vi "WaitForMoveComplete.vi"(6 "timeout (5000 ms)":i32=5000, 8 "error in (no error)":errorcluster, 11 "XYStage":refnum<class "XYStage.lvclass">) -> (0 "error out":errorcluster, 2 "move complete":bool, 3 "XYStage out":refnum<class "XYStage.lvclass">)   [LabVIEW 2013, in "XYStage.lvclass"]
doc: "---------------------------------------------------------------\nJKI State Machine Objects™\nhttp://jki.net/state-machine-objects/\nCopyright (C) 2005-2015, JKI <info@jki.net>\nALL RIGHTS RESERVEDJKI State Machine Objects (SMO) 1.0.0.4\nJKI - JKI\nCopyright (c) 2015, JKI"
uses:
  XYStage.lvclass
  <vilib>/JKI/JKI SMO/SMO/SMO.lvclass
  <vilib>/JKI/JKI SMO/SMO/Typedefs/SMOState --Enum.ctl
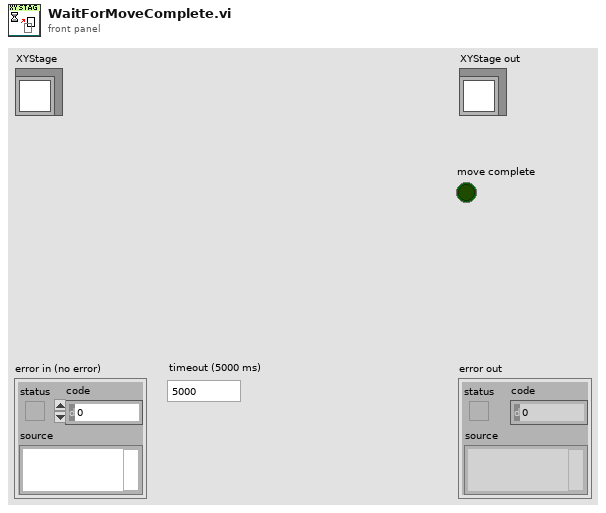
[diagram p1: front panel]
types:
  T1 = typedef "SMO.lvclass/Protected Events.ctl" = cluster{"StopProcesses":refnum<user-event>, "AbortProcesses":refnum<user-event>, "Config Changed":refnum<user-event>}
  T2 = typedef "SMO.lvclass/Public Events.ctl" = cluster{"Error":refnum<user-event>, "State":refnum<user-event>}
  T3 = typedef "XYStage.lvclass/PublicEvents--Cluster.ctl" = cluster{"MoveComplete":refnum<user-event>, "NewPosition":refnum<user-event>, "UpdatedNamedPosition":refnum<user-event>, "MoveStarted":refnum<user-event>}
  T4 = typedef "SMO.lvclass/SMOState --Enum.ctl" = enum16{"unknown", "Created", "Started", "Stopped"}
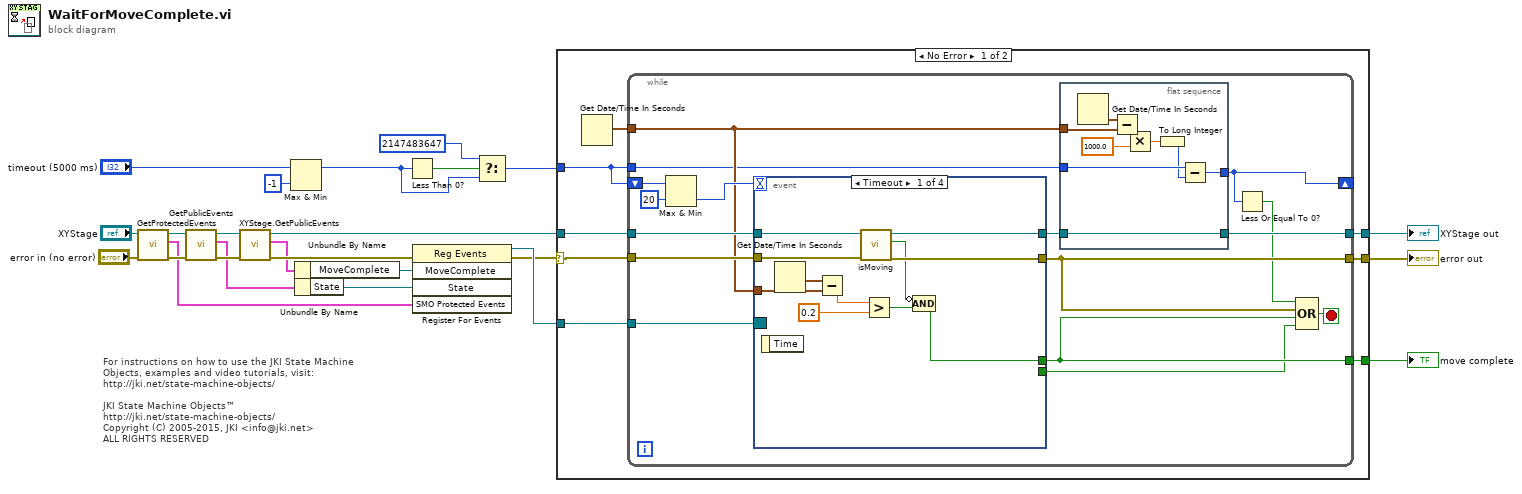
[diagram p0: block diagram]
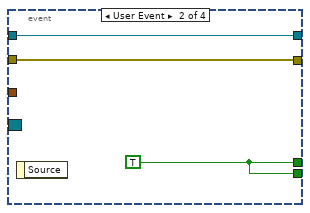
[diagram p2: hidden frame]
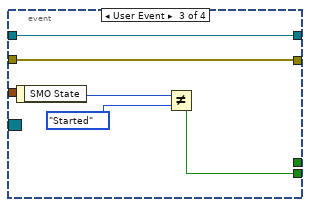
[diagram p3: hidden frame]
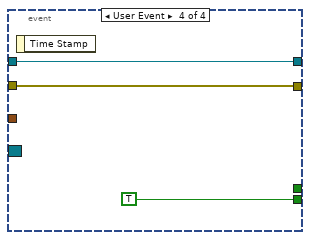
[diagram p4: hidden frame]
diagram:
  # "For instructions on how to use the JKI State Machine Objects, examples and video tutorials, visit:\nhttp://jki.net/state-machine-objects/\n\nJKI State Machine Objects™\nhttp://jki.net/state-machine-objects/\nCopyright (C) 2005-2015, JKI <info@jki.net>\nALL RIGHTS RESERVED"
  n1 = call <vilib>:"GetProtectedEvents.vi"("error in (no error)"="error in (no error)", "SMO"="XYStage") -> ("error out"=w2:errorcluster, "SMO Protected Events"=w1:T1, "SMO out"=w4:refnum<class "XYStage.lvclass">)  [unwired: 7 in]
  n2 = call <vilib>:"GetPublicEvents.vi"("error in (no error)"=w2, "SMO"=w4) -> ("error out"=w12:errorcluster, "Public Events"=w11:T2, "SMO out"=w13:refnum<class "XYStage.lvclass">)  [unwired: 7 in]
  n3 = call "XYStage.GetPublicEvents.vi"("error in (no error)"=w12, "XYStage"=w13) -> ("error out"=w20:errorcluster, "XYStage Public Events"=w19:T3, "XYStage out"=w14:refnum<class "XYStage.lvclass">)  [unwired: 7 in]
  n4 = Max & Min(x="timeout (5000 ms)", y=-1) -> (max(x,y)=w8:i32)  [unwired: 1 out]
  n5 = Unbundle By Name(w19) -> ("MoveComplete"=w18:refnum<user-event>)
  n6 = Unbundle By Name(w11) -> ("State"=w10:refnum<user-event>)
  n7 = Less Than 0?(x=w8) -> (x < 0?=w9:bool)
  n8 = register-events(error in=w20, w18, w10, w1) -> (reference out=w17:refnum<event-registration>, error out=w15:errorcluster)  [unwired: 1 in]
  n9 = Select(t=2147483647 ("y"), s=w9, f=w8) -> (s? t:f=w7:i32)
  n10 = case shown="No Error" w15 {
    selector: w15 -> [w29 w80]
    tunnel: w17 -> [w32 _]
    tunnel: w7 -> [w25 _]
    tunnel: [w31 _] -> w23
    tunnel: w14 -> [w30 w81]
    tunnel: [w28 w81] -> w22
    tunnel: [w27 w80] -> w21
    frame No Error {
      n11 = Get Date/Time In Seconds() -> (seconds since 1Jan1904=w26:timestamp)
      n12 = while {
        tunnel: w32 -> [w48]
        tunnel: [w44] -> w31
        tunnel: w30 -> [w47]
        tunnel: w29 -> [w46]
        tunnel: [w36] -> w28
        tunnel: [w45] -> w27
        tunnel: w26 -> [w38]
        shift-right: [w34] -> _
        shift-left: w25 -> [w41]
        tunnel: w25 -> [w35]
        stop <- w43 stop-if-true
        n13 = Max & Min(x=w41, y=20) -> (min(x,y)=w39:i32)  [unwired: 1 out]
        n14 = event shown="[0] Timeout" {
          selector: w48 -> [_ _ _ _]
          dyn-events: _ -> [_ _ _ _]
          timeout: w39 -> [_ _ _ _]
          tunnel: [w58 w71 _ _] -> w44
          tunnel: [_ w71 w74 TRUE] -> w42
          tunnel: w47 -> [w63 w70 w73 w79]
          tunnel: w46 -> [w68 w69 w72 w78]
          tunnel: [w67 w70 w73 w79] -> w37
          tunnel: [w66 w69 w72 w78] -> w45
          tunnel: w38 -> [w65 _ _ _]
          event Timeout {
            n15 = event-data() -> ()  [unwired: 1 in, 1 out]
            n16 = Get Date/Time In Seconds() -> (seconds since 1Jan1904=w64:timestamp)
            n17 = Subtract(x=w64, y=w65) -> (x-y=w62:dbl)
            n18 = call "isMoving.vi"("error in (no error)"=w68, "XYStage"=w63) -> ("error out"=w66:errorcluster, "Moving"=w59:bool, "XYStage out"=w67:refnum<class "XYStage.lvclass">)  [unwired: 7 in]
            n19 = Greater?(x=w62, y=0.2) -> (0:w60:bool)
            n20 = Compound Arithmetic op=AND(invert w59, w60) -> (w58:bool)
          }
          event User Event {
            w71 = TRUE
            n21 = event-data() -> ()  [unwired: 1 in, 1 out]
          }
          event User Event {
            n22 = event-data() -> ("SMO State"=w76:T4)  [unwired: 1 in]
            n23 = Not Equal?(x=w76, y=SMOState_--Enum."Started") -> (x != y?=w74:bool)
          }
          event User Event {
            n24 = event-data() -> ()  [unwired: 1 in, 1 out]
          }
        }
        n25 = flat-sequence {
          tunnel: w38 -> [w55]
          tunnel: w37 -> [w57]
          tunnel: [w57] -> w36
          tunnel: w35 -> [w51]
          tunnel: [w49] -> w34
          frame #0 {
            n26 = Get Date/Time In Seconds() -> (seconds since 1Jan1904=w56:timestamp)
            n27 = Subtract(x=w56, y=w55) -> (x-y=w54:dbl)
            n28 = Multiply(x=w54, y=1000.0) -> (x*y=w52:dbl)
            n29 = To Long Integer(number=w52) -> (32bit integer=w50:i32)
            n30 = Subtract(x=w51, y=w50) -> (x-y=w49:i32)
          }
        }
        n31 = Less Or Equal To 0?(x=w34) -> (x <= 0?=w33:bool)
        n32 = Compound Arithmetic op=OR(w33, w45, w44, w42) -> (w43:bool)
      }
    }
    frame Error {
    }
  }
  "error out" <- w21
  "XYStage out" <- w22
  "move complete" <- w23
